vi "temp chart display calculations.vi"(0 "power in (0-1)":dbl format="%.2f", 2 "Mode":enum16{"Expanded", "Shrunk"}(ring), 5 "temp in":dbl format="%.2f", 7 "Control Parameters":T2={"Setpoint"=50.0, "Control bandwidth"=4.0, "Settle bandwidth"=1.0, "Integral time"=30.0, "Int\non"=TRUE, "Derivative time"=0.5, "Der\non"=TRUE, "Settle time"=200.0} {"Settle time" format="%.2f"; "Derivative time" format="%.2f"; "Integral time" format="%.2f"; "Settle bandwidth" format="%.2f"; "Control bandwidth" format="%.2f"; "Setpoint" format="%.2f"}, 9 "Scale Control In":T1, 11 "Temp History in":refnum<vi>, 13 "range indicator refs":T4) -> (4 "Setpoint out":dbl format="%.2f", 6 "Temperature History out":T3 {"?" format="%.2f"; "?" format="%.2f"; "?" format="%.2f"; "?" format="%.2f"; "?" format="%.2f"; "?" format="%.2f"; "temp out" format="%.2f"}, 10 "Scale Control Out":T1, 14 "range indicators out":T5)   [LabVIEW 2016]
doc: "this vi does all of the calculations an manipulations necessary for the temp chart display including normalizing the power out to the current scale\n\nPaul K Dixon\nPhysics 350\nCSUSB Physics"
uses:
  typedefs/status indicator.ctl
  typedefs/scale control.ctl
  typedefs/control parameters.ctl
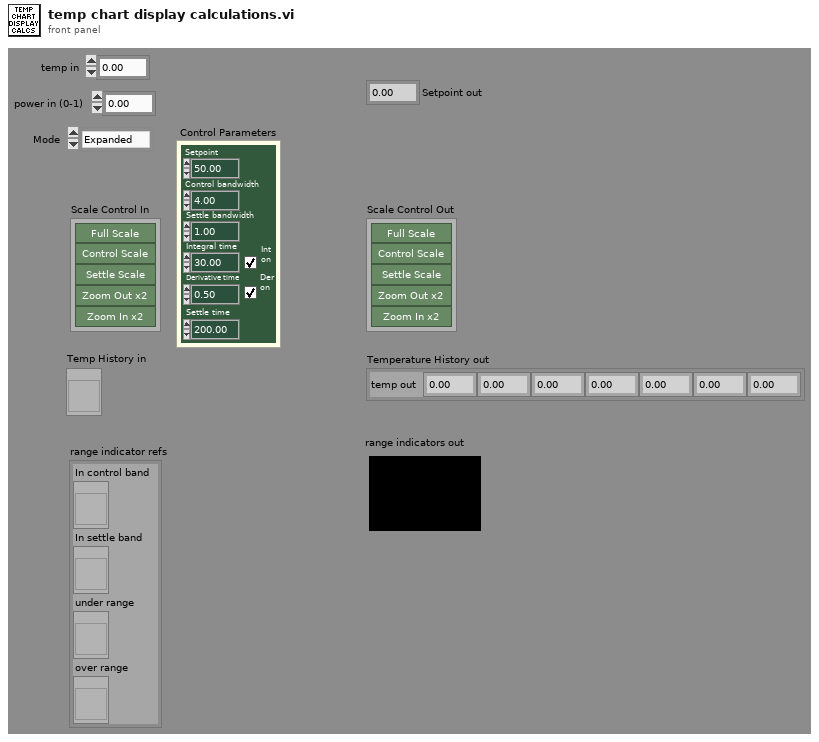
[diagram p1: front panel]
types:
  T1 = typedef "scale control.ctl" = cluster{"Full Scale":bool, "Control Scale":bool, "Settle Scale":bool, "Zoom Out":bool, "Zoom In":bool}
  T2 = typedef "control parameters.ctl" = cluster{"Setpoint":dbl, "Control bandwidth":dbl, "Settle bandwidth":dbl, "Integral time":dbl, "Int\non":bool, "Derivative time":dbl, "Der\non":bool, "Settle time":dbl}
  T3 = cluster{"temp out":dbl, dbl, dbl, dbl, dbl, dbl, dbl}
  T4 = cluster{"In control band":refnum<vi>, "In settle band":refnum<vi>, "under range":refnum<vi>, "over range":refnum<vi>}
  T5 = typedef "status indicator.ctl" = cluster{"In control band":bool, "In settle band":bool, "under range":bool, "over range":bool}
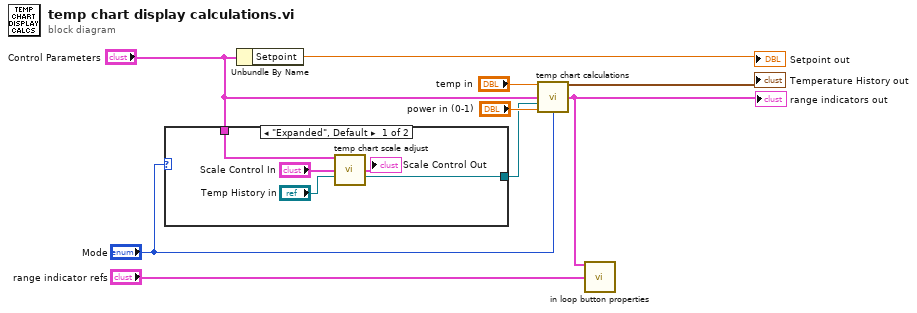
[diagram p0: block diagram]
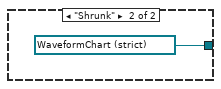
[diagram p2: hidden frame]
diagram:
  n1 = case shown="\"Expanded\", Default" "Mode" {
    tunnel: [w13 refnum<vi> refnum ("Temperature History out")] -> w5
    tunnel: "Control Parameters" -> [w12 _]
    frame "Expanded", Default {
      n2 = call "temp chart scale adjust.vi"("Control Parameters"=w12, "Scale Control In"="Scale Control In", "Temperature History in"="Temp History in") -> ("Scale Control Out"=→"Scale Control Out":T1, "Temperature History out"=w13:refnum<vi>)  [unwired: 1 in, 10 out]
    }
    frame "Shrunk" {
    }
  }
  n3 = Unbundle By Name("Control Parameters") -> ("Setpoint"=→"Setpoint out":dbl)
  n4 = call "temp chart calculations.vi"("temp in"="temp in", "Control Parameters"="Control Parameters", "Temperature History in"=w5, "norm power in"="power in (0-1)", "Mode"="Mode") -> ("Temperature History"=→"Temperature History out":T3, "range indicators"=w1:T5)  [unwired: 9 out]
  "range indicators out" <- w1
  n5 = call "in loop button properties.vi"("range settings"=w1, "range indicator refs"="range indicator refs") -> ()  [unwired: 1 in, 13 out]
